vi "BRig_dataTrial_Cue2_iTrial_1A.vi"() -> (2 "output_Cue2_iTrial_1A":i32)   [LabVIEW 2014]
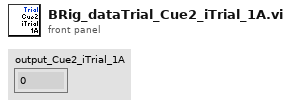
[diagram p1: front panel]
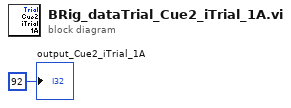
[diagram p0: block diagram]
diagram:
  "output_Cue2_iTrial_1A" <- 92 ("output_iBlock")
